vi "数据处理整合 (子VI).vi"() -> (3 "已排序的数组":string[](array[string]))   [LabVIEW 2016]
uses:
  <userlib>/_OpenG.lib/array/array.llb/Remove Duplicates from 1D Array (String)__ogtk.vi
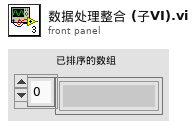
[diagram p1: front panel]
types:
  T1 = cluster{"PH":string[][], "CODCr":string[][], "氨氮":string[][], "CODMn":string[][], "总氮":string[][], "总磷":string[][], "电导率":string[][], "水温":string[][], "DO":string[][], "浊度":string[][], "叶绿素":string[][], "藻密度":string[][]}
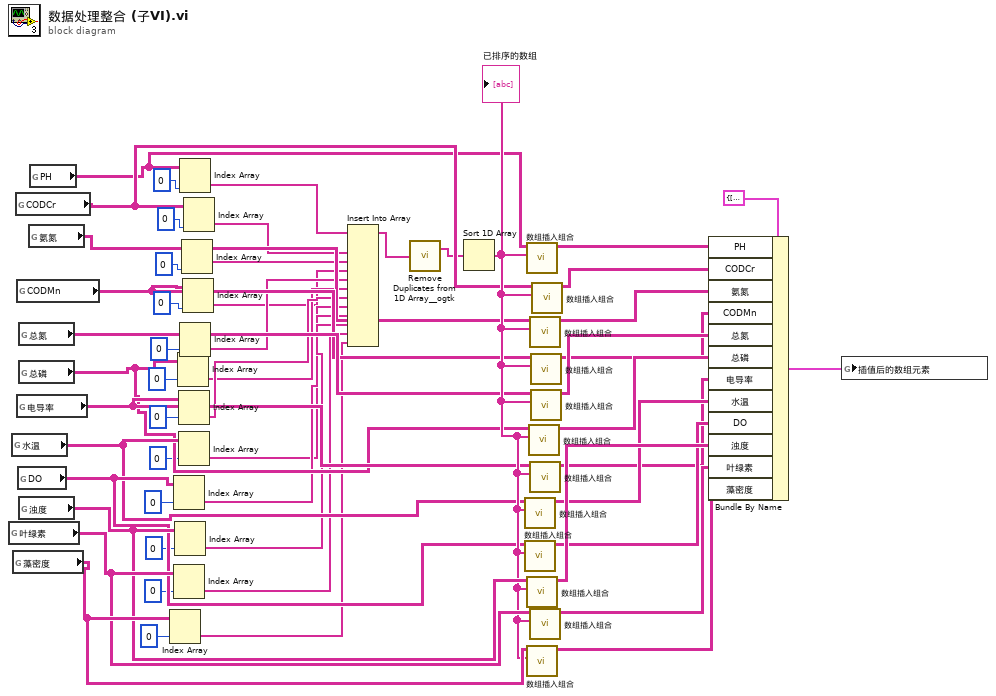
[diagram p0: block diagram]
diagram:
  n1 = global read "全局 所有参数.vi" "叶绿素"() -> (w41:string[][])
  n2 = global read "全局 所有参数.vi" "水温"() -> (w37:string[][])
  n3 = global read "全局 所有参数.vi" "藻密度"() -> (w42:string[][])
  n4 = global read "全局 所有参数.vi" "CODCr"() -> (w31:string[][])
  n5 = global read "全局 所有参数.vi" "CODMn"() -> (w33:string[][])
  n6 = global read "全局 所有参数.vi" "电导率"() -> (w36:string[][])
  n7 = global read "全局 所有参数.vi" "DO"() -> (w38:string[][])
  n8 = global read "全局 所有参数.vi" "总氮"() -> (w34:string[][])
  n9 = global read "全局 所有参数.vi" "总磷"() -> (w35:string[][])
  n10 = global read "全局 所有参数.vi" "浊度"() -> (w40:string[][])
  n11 = global read "全局 所有参数.vi" "氨氮"() -> (w32:string[][])
  n12 = global read "全局 所有参数.vi" "PH"() -> (w27:string[][])
  n13 = Index Array(array=w42, index (col)=0 ("索引 (行)")) -> (element=w25:string[])  [unwired: 1 in]
  n14 = Index Array(array=w38, index (col)=0 ("索引 (行)")) -> (element=w22:string[])  [unwired: 1 in]
  n15 = Index Array(array=w41, index (col)=0 ("索引 (行)")) -> (element=w24:string[])  [unwired: 1 in]
  n16 = Index Array(array=w40, index (col)=0 ("索引 (行)")) -> (element=w23:string[])  [unwired: 1 in]
  n17 = Index Array(array=w35, index (col)=0 ("索引 (行)")) -> (element=w19:string[])  [unwired: 1 in]
  n18 = Index Array(array=w36, index (col)=0 ("索引 (行)")) -> (element=w20:string[])  [unwired: 1 in]
  n19 = Index Array(array=w37, index (col)=0 ("索引 (行)")) -> (element=w21:string[])  [unwired: 1 in]
  n20 = Index Array(array=w27, index (col)=0 ("索引 (行)")) -> (element=w14:string[])  [unwired: 1 in]
  n21 = Index Array(array=w34, index (col)=0 ("索引 (行)")) -> (element=w18:string[])  [unwired: 1 in]
  n22 = Index Array(array=w32, index (col)=0 ("索引 (行)")) -> (element=w16:string[])  [unwired: 1 in]
  n23 = Index Array(array=w33, index (col)=0 ("索引 (行)")) -> (element=w17:string[])  [unwired: 1 in]
  n24 = Index Array(array=w31, index (col)=0 ("索引 (行)")) -> (element=w15:string[])  [unwired: 1 in]
  n25 = Insert Into Array(array=w14, new element #1=w15, new element #2=w16, new element #3=w17, new element #4=w18, new element #5=w19, new element #6=w20, new element #7=w21, new element #8=w22, new element #9=w23, new element #10=w24, new element #11=w25) -> (w26:string[])  [unwired: 1 in]
  n26 = call-poly <userlib>:"Remove Duplicates from 1D Array__ogtk.vi"("Input Array"=w26) -> ("Output Array"=w13:string[])  [unwired: 1 out]
  n27 = Sort 1D Array(array=w13) -> (sorted array=w39:string[])
  "已排序的数组" <- w39
  n28 = call "数组插入组合.vi"("排序后的一维数组"=w39, "输入数组"=w37) -> ("输出结果"=w49:string[][])  [unwired: 9 in]
  n29 = call "数组插入组合.vi"("排序后的一维数组"=w39, "输入数组"=w38) -> ("输出结果"=w50:string[][])  [unwired: 9 in]
  n30 = call "数组插入组合.vi"("排序后的一维数组"=w39, "输入数组"=w27) -> ("输出结果"=w30:string[][])  [unwired: 9 in]
  n31 = call "数组插入组合.vi"("排序后的一维数组"=w39, "输入数组"=w40) -> ("输出结果"=w51:string[][])  [unwired: 9 in]
  n32 = call "数组插入组合.vi"("排序后的一维数组"=w39, "输入数组"=w42) -> ("输出结果"=w53:string[][])  [unwired: 9 in]
  n33 = call "数组插入组合.vi"("排序后的一维数组"=w39, "输入数组"=w35) -> ("输出结果"=w47:string[][])  [unwired: 9 in]
  n34 = call "数组插入组合.vi"("排序后的一维数组"=w39, "输入数组"=w32) -> ("输出结果"=w44:string[][])  [unwired: 9 in]
  n35 = call "数组插入组合.vi"("排序后的一维数组"=w39, "输入数组"=w36) -> ("输出结果"=w48:string[][])  [unwired: 9 in]
  n36 = call "数组插入组合.vi"("排序后的一维数组"=w39, "输入数组"=w41) -> ("输出结果"=w52:string[][])  [unwired: 9 in]
  n37 = call "数组插入组合.vi"("排序后的一维数组"=w39, "输入数组"=w33) -> ("输出结果"=w45:string[][])  [unwired: 9 in]
  n38 = call "数组插入组合.vi"("排序后的一维数组"=w39, "输入数组"=w34) -> ("输出结果"=w46:string[][])  [unwired: 9 in]
  n39 = call "数组插入组合.vi"("排序后的一维数组"=w39, "输入数组"=w31) -> ("输出结果"=w43:string[][])  [unwired: 9 in]
  n40 = Bundle By Name(cluster=T1 {"PH"=[], "CODCr"=[], "氨氮"=[], "CODMn"=[], "总氮"=[], "总磷"=[], "电导率"=[], "水温"=[], "DO"=[], "浊度"=[], "叶绿素"=[], "藻密度"=[]} ("插值后的数组元素"), "PH"=w30, "CODCr"=w43, "氨氮"=w44, "CODMn"=w45, "总氮"=w46, "总磷"=w47, "电导率"=w48, "水温"=w49, "DO"=w50, "浊度"=w51, "叶绿素"=w52, "藻密度"=w53) -> (w29:T1)
  n41 = global write "插值后的新数组.vi" "插值后的数组元素"(w29) -> ()
